vi "Destroy.vi"(8 "error in (no error)":errorcluster, 11 "StringMap in":refnum<class "StringMap.lvclass">) -> (0 "error out":errorcluster, 5 "MapImp out":refnum<class "MapImp.lvclass">, 7 "StringMap out":refnum<class "StringMap.lvclass">)   [LabVIEW 2013, in "LapDog.Collections.v1.Maps.lvlib" / "StringMap.lvclass"]
doc: "Add a key-value pair to the map.\n\nIf the key already exists, error 510202 is returned."
uses:
  StringMap.lvclass
  MapImp/MapImp.lvclass
  StringMap.lvclass/StringMap.ctl
  ObjectMap/ObjectMap.lvclass
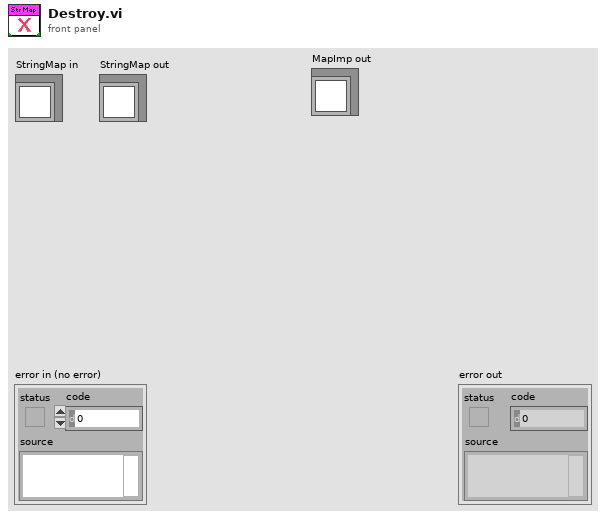
[diagram p1: front panel]
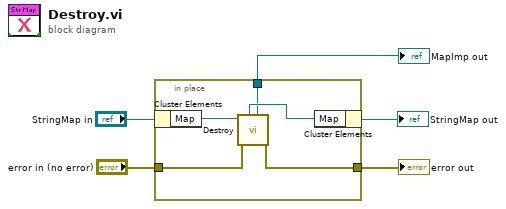
[diagram p0: block diagram]
diagram:
  n1 = in-place {
    in-place-border: [w8] -> w3
    in-place-border: "error in (no error)" -> [w7]
    in-place-border: [w6] -> w1
    n2 = in-place-cluster #1("StringMap in") -> ("Map"=w10:refnum<class "ObjectMap.lvclass">)
    n3 = call-dynamic "Destroy.vi"("error in (no error)"=w7, "Map in"=w10) -> ("error out"=w6:errorcluster, "MapImp out"=w8:refnum<class "MapImp.lvclass">, "Map out"=w9:refnum<class "ObjectMap.lvclass">)  [unwired: 7 in]
    n4 = in-place-cluster #1("Map"=w9) -> (→"StringMap out":refnum<class "StringMap.lvclass">)
  }
  "error out" <- w1
  "MapImp out" <- w3
